vi "LinxSpiWriteRead.vi"(5 "CS Configuration":T1, 7 "SPI Channel":u8, 8 "Error In":errorcluster, 9 "SPI Frame Size (0)":u8, 10 "Data":u8[](array[numeric]), 11 "LINX Resource":T3) -> (0 "Error Out":errorcluster, 2 "Data":u8[](array[numeric]), 3 "LINX Resource":T3, 4 "status":i32)   [LabVIEW 2019, in "LMH-LINX.lvlib" / "Local IO.lvlib"]
uses:
  <vilib>/MakerHub/LINX/Private/Local IO/Local IO.lvlib
  <vilib>/MakerHub/LINX/Private/Type Defs/LINX Ref.ctl
  <vilib>/MakerHub/LINX/Private/Type Defs/Platform.ctl
  <vilib>/MakerHub/LINX/Private/Type Defs/Interface.ctl
  <vilib>/MakerHub/LINX/Private/Device/Type Defs/LINX Device Config.ctl
  <vilib>/MakerHub/LINX/Private/Device/Type Defs/TCP Config.ctl
  <vilib>/MakerHub/LINX/Private/Device/Type Defs/Channels.ctl
  <vilib>/MakerHub/LINX/Public/Peripherals/SPI/SPI CS Config.ctl
  <vilib>/MakerHub/LINX/Private/Type Defs/Peripherals/SPI/SPI CS Logic Level.ctl
  <vilib>/MakerHub/LINX/Private/Type Defs/Error Type.ctl
  <vilib>/MakerHub/LINX/LMH-LINX.lvlib
  <vilib>/MakerHub/LINX/Private/Type Defs/Channel FGV States.ctl
  <vilib>/myRIO/Common/Instrument Driver Framework/myRIO v1.0/SPI/typedefs/SPI Frame Length.ctl
  <vilib>/myRIO/Common/Instrument Driver Framework/myRIO v1.0/SPI/typedefs/SPI Data Direction.ctl
  <vilib>/myRIO/Common/Instrument Driver Framework/myRIO v1.0/SPI/typedefs/SPI Clock Polarity.ctl
  <vilib>/myRIO/Common/Instrument Driver Framework/myRIO v1.0/SPI/typedefs/SPI Clock Phase.ctl
  <vilib>/myRIO/Instrument Drivers/Onboard IO/SPI/typedefs/SPI Configuration.ctl
  <vilib>/myRIO/Common/Instrument Driver Framework/myRIO v1.0/SPI/typedefs/SPI Channels Enum.ctl
  <vilib>/myRIO/Common/Instrument Driver Framework/Utilities/typedefs/Generic FPGA Reference.ctl
  <vilib>/myRIO/Common/Instrument Driver Framework/Utilities/typedefs/myRIO v1.0 Reference.ctl
  <vilib>/myRIO/Common/Instrument Driver Framework/Utilities/typedefs/Hardware Version Enum.ctl
  <vilib>/myRIO/Common/Instrument Driver Framework/Utilities/typedefs/myRIO Generic Hardware Reference.ctl
  <vilib>/myRIO/Instrument Drivers/Onboard IO/SPI/typedefs/SPI Reference.ctl
  <vilib>/MakerHub/LINX/Resources/liblinxdevice.dll
  <vilib>/MakerHub/LINX/Private/Device/Device.lvlib
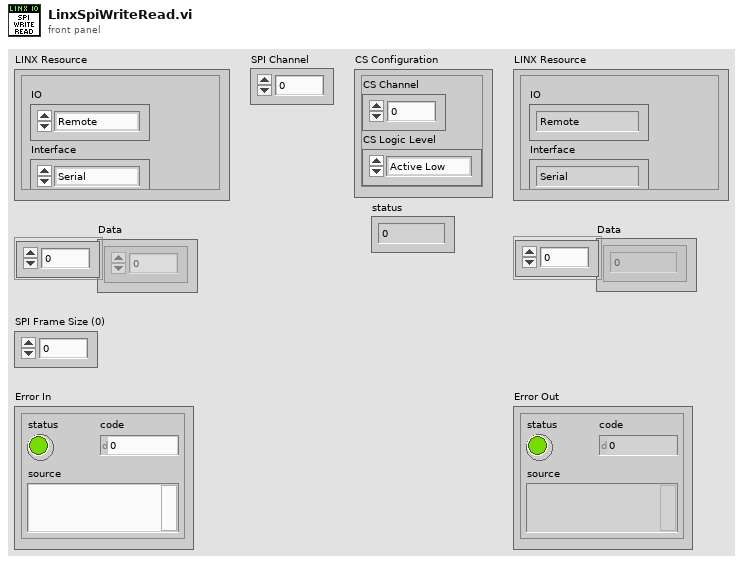
[diagram p1: front panel]
types:
  T1 = typedef "LMH-LINX.lvlib/SPI CS Config.ctl" = cluster{"CS Channel":u8, "CS Logic Level":T2}
  T2 = typedef "LMH-LINX.lvlib/SPI CS Logic Level.ctl" = enum8{"Active Low", "Active High"}
  T3 = typedef "LMH-LINX.lvlib/LINX Ref.ctl" = cluster{"IO":T4, "Interface":T5, "LINX Device Config":T6}
  T4 = typedef "LMH-LINX.lvlib/Platform.ctl" = enum16{"Remote", "Local"}
  T5 = typedef "LMH-LINX.lvlib/Interface.ctl" = enum16{"Serial", "TCP"}
  T6 = typedef "LMH-LINX.lvlib/Device.lvlib/LINX Device Config.ctl" = cluster{"Interface":T5, "COM Port":refnum<visa-resource-name>, "TCP Configuration":T7, "Device Family":u8, "Device ID":u8, "Device Name":string, "TCP Ref":refnum<k5>, "Channels":T8}
  T7 = typedef "LMH-LINX.lvlib/Device.lvlib/TCP Config.ctl" = cluster{"IP Address":string, "Port":u16}
  T8 = typedef "LMH-LINX.lvlib/Channels.ctl" = cluster{"DI":u8[], "DO":u8[], "AI":u8[], "AO":u8[], "PWM":u8[], "QE":u8[], "UART":u8[], "I2C 2":u8[], "SPI":u8[], "CAN":u8[], "Servo":u8[], "AI Ref (V)":dbl, "AI Resolution (Bits)":u8, "AO Ref (V)":dbl, "AO Resolution (Bits)":u8}
  T9 = typedef "LMH-LINX.lvlib/Error Type.ctl" = enum16{"Unknown", "Timeout", "Corrupt Return Packet", "Unable To Connect", "Command Not Supported", "Channel DNE", "Invalid COM Config", "Firmware Version Mismatch", "myRIO Support", "CMD Specific Error", "Local IO Not Supported"}
  T10 = typedef "LMH-LINX.lvlib/Channel FGV States.ctl" = enum16{"Initialize", "Get", "Set"}
  T11 = typedef "SPI.lvlib/SPI Reference.ctl" = cluster{"myRIO Reference":T12, "SPI Channels Enum":T16, "SPI Configuration":T17}
  T12 = typedef "myRIO Generic Hardware Reference.ctl" = cluster{"myRIO Model":T13, "myRIO Hardware Reference":T14}
  T13 = typedef "Hardware Version Enum.ctl" = enum16{"Unknown", "myRIO-1900", "myRIO-1950"}
  T14 = typedef "myRIO v1.0 Reference.ctl" = cluster{"Generic FPGA Reference":T15, "Allow multiple opens":bool}
  T15 = typedef "Generic FPGA Reference.ctl" = refnum<k20>
  T16 = typedef "SPI Channels Enum.ctl" = enum16{"Not Connected", "A/SPI", "B/SPI"}
  T17 = typedef "SPI.lvlib/SPI Configuration.ctl" = cluster{"Frequency [Hz]":dbl, "Clock Phase":T18, "Clock Polarity":T19, "Data Direction":T20, "Frame Length":T21}
  T18 = typedef "SPI Clock Phase.ctl" = enum8{"Leading", "Trailing"}
  T19 = typedef "SPI Clock Polarity.ctl" = enum8{"Low", "High"}
  T20 = typedef "SPI Data Direction.ctl" = enum8{"Most significant bit first", "Least significant bit first"}
  T21 = typedef "SPI Frame Length.ctl" = u8
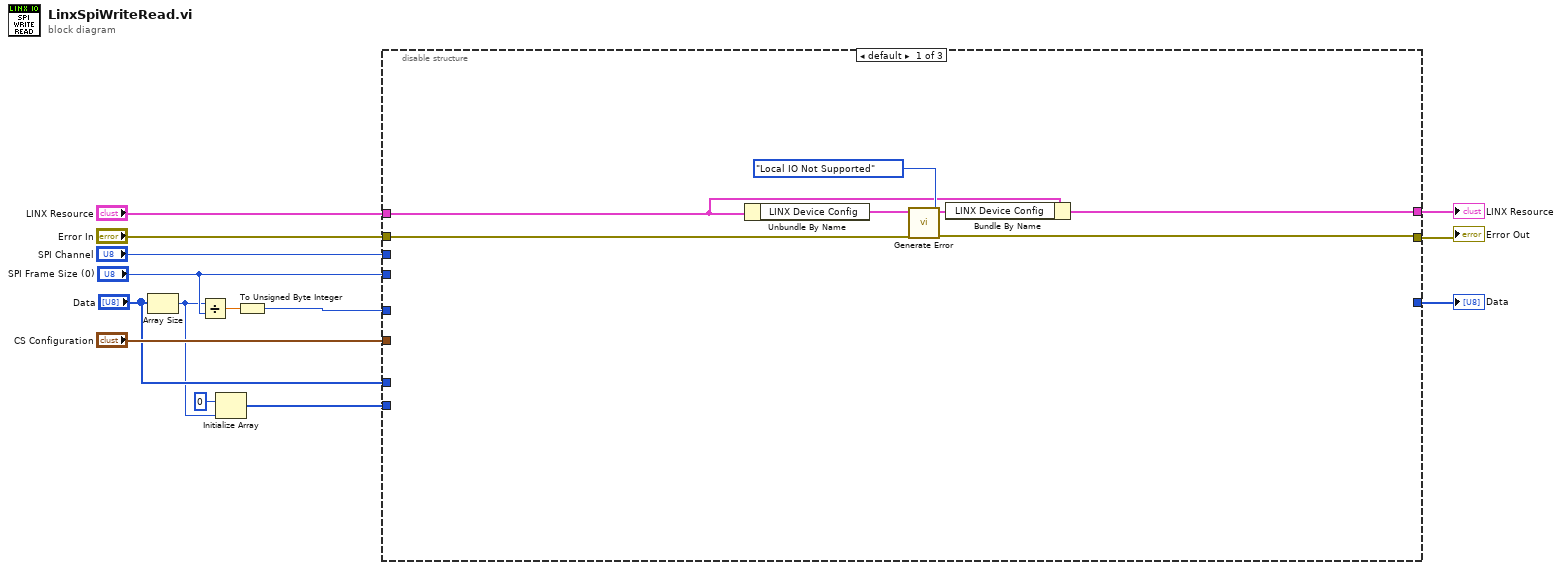
[diagram p0: block diagram]
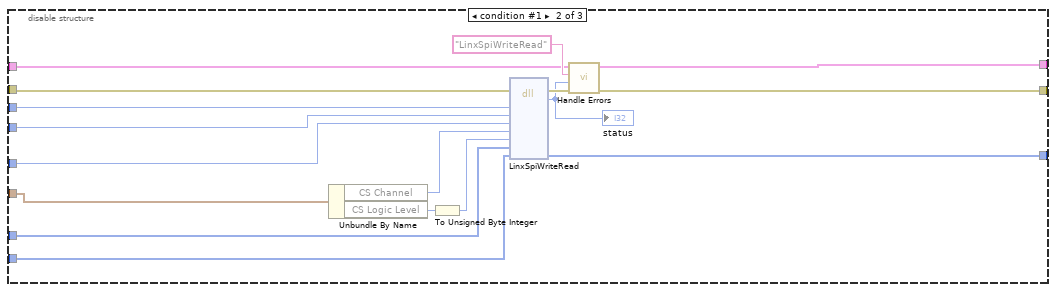
[diagram p2: hidden frame]
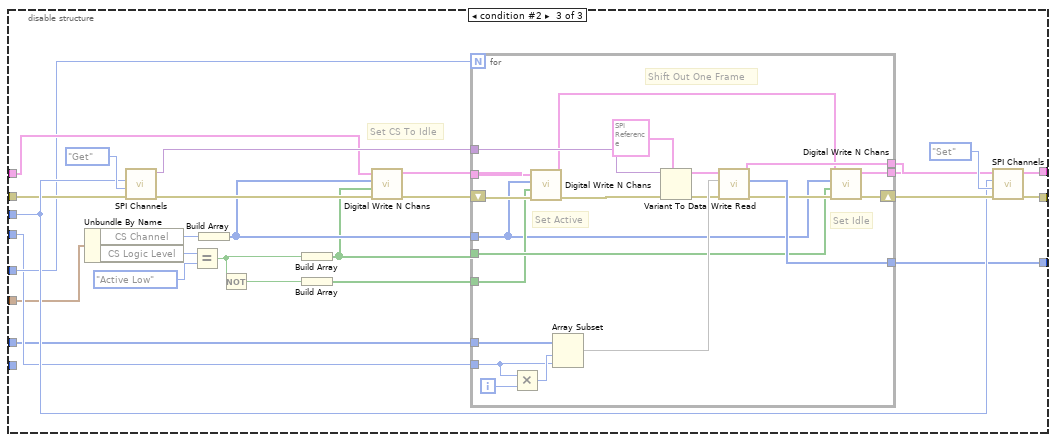
[diagram p3: hidden frame]
diagram:
  n1 = Array Size(array="Data") -> (size(s)=w4:i32)
  n2 = Divide(x=w4, y="SPI Frame Size (0)") -> (x/y=w7:dbl)
  n3 = Initialize Array(u8 0 ("element"), w4) -> (w2:u8[])
  n4 = To Unsigned Byte Integer(number=w7) -> (unsigned 8bit integer=w6:u8)
  n5 = disable-structure shown="default" {
    disable-tunnel: [w16 w23 w41] -> w14
    disable-tunnel: "LINX Resource" -> [w18 w33 w48]
    disable-tunnel: "Error In" -> [w20 w36 w49]
    disable-tunnel: "SPI Channel" -> [_ w34 w50]
    disable-tunnel: [w15 w24 w40] -> w10
    disable-tunnel: "SPI Frame Size (0)" -> [_ w32 w46]
    disable-tunnel: w6 -> [_ w30 w47]
    disable-tunnel: "CS Configuration" -> [_ w31 w44]
    disable-tunnel: "Data" -> [_ w26 w45]
    disable-tunnel: w2 -> [_ w25 _]
    disable-tunnel: [_ w22 w39] -> w1
    frame condition #0 (active) {
      n6 = Unbundle By Name(w18) -> ("LINX Device Config"=w19:T6)
      n7 = call <vilib>:"Generate Error.vi"("Error In"=w20, "Error Type"=Error_Type."Local IO Not Supported", "LINX Device Config"=w19) -> ("Error Out"=w15:errorcluster, "Dup LINX Device Config"=w17:T6)  [unwired: 7 in]
      n8 = Bundle By Name(cluster=w18, "LINX Device Config"=w17) -> (w16:T3)
    }
    frame condition #1 {
      n9 = Unbundle By Name(w31) -> ("CS Channel"=w29:u8, "CS Logic Level"=w28:T2)
      n10 = To Unsigned Byte Integer(number=w28) -> (unsigned 8bit integer=w27:u8)
      n11 = dll-call lib="E:/lv2019/dist/vi.lib/MakerHub/LINX/Resources/liblinxdevice.*" fn="LinxSpiWriteRead"(error in=w36, "channel"=w34, "frameSize"=w32, "numFrames"=w30, "csChan"=w29, "csLL"=w27, "sendBuffer"=w26, "recBuffer"=w25) -> (error out=w37:errorcluster, "status"=w35:i32, "recBuffer"=w22:u8[])  [unwired: 8 in, 1 out]
      "status" <- w35
      n12 = call <vilib>:"Handle Errors.vi"("Error In"=w37, "LinxStatus"=w35, "Function Name"="LinxSpiWriteRead", "LINX Resource"=w33) -> ("Error Out"=w24:errorcluster, "LINX Resource"=w23:T3)  [unwired: 6 in]
    }
    frame condition #2 {
      # "Set CS To Idle"
      n13 = Unbundle By Name(w44) -> ("CS Channel"=w43:u8, "CS Logic Level"=w42:T2)
      n14 = call <vilib>:"SPI Channels.vi"("Error In"=w49, "Channel State"=Channel_FGV_States."Get", "Channel Number"=w50) -> ("Error Out"=w59:errorcluster, "SPI Channel"=w60:variant)  [unwired: 7 in]
      n15 = Equal?(x=w42, y=SPI_CS_Logic_Level."Active Low") -> (x = y?=w54:bool)
      n16 = Build Array(w43) -> (w55:u8[])
      n17 = Not(x=w54) -> (.not. x?=w52:bool)
      n18 = Build Array(w54) -> (w53:bool[])
      n19 = Build Array(w52) -> (w51:bool[])
      n20 = call <vilib>:"Digital Write N Chans.vi"("Error In"=w59, "Values"=w53, "DO Channels"=w55, "LINX Resource"=w48) -> ("Error Out"=w58:errorcluster, "LINX Resource"=w56:T3)  [unwired: 6 in]
      n21 = for {
        N: w47 -> [_]
        tunnel: [w85] -> w61
        tunnel: w60 -> [w84]
        tunnel: w45 -> [w82]
        tunnel: [w83] -> w39
        shift-right: [w74] -> w62
        shift-left: w58 -> [w77]
        tunnel: w46 -> [w78]
        tunnel: w56 -> [w75]
        tunnel: w55 -> [w68]
        tunnel: [w71] -> w41
        tunnel: w53 -> [w70]
        tunnel: w51 -> [w69]
        i -> [w80]
        # "Set Idle"
        # "Shift Out One Frame"
        # "Set Active"
        n22 = Multiply(x=w78, y=w80) -> (x*y=w79:i32)
        n23 = call <vilib>:"Digital Write N Chans.vi"("Error In"=w77, "Values"=w69, "DO Channels"=w68, "LINX Resource"=w75) -> ("Error Out"=w76:errorcluster, "LINX Resource"=w72:T3)  [unwired: 6 in]
        n24 = Array Subset(array=w82, index=w79, length=w78) -> (w81:u8[])
        n25 = Variant To Data(error in=w76, type=T11 {"myRIO Reference"={"myRIO Model"=enum."Unknown", "myRIO Hardware Reference"={"Generic FPGA Reference"=refnum, "Allow multiple opens"=FALSE}}, "SPI Channels Enum"=enum."Not Connected", "SPI Configuration"={"Frequency [Hz]"=0.0, "Clock Phase"=enum."Leading", "Clock Polarity"=enum."Low", "Data Direction"=enum."Most significant bit first", "Frame Length"=8}} ("SPI Ref In"), Variant=w84) -> (data=w66:T11, error out=w65:errorcluster)
        n26 = call <vilib>:"Write Read.vi"("error in (no error)"=w65, "Frames to Write"=w81, "SPI Ref In"=w66) -> ("error out"=w73:errorcluster, "Frames Read"=w83:u16[], "SPI Ref Out"=w85:T11)  [unwired: 6 in]
        n27 = call <vilib>:"Digital Write N Chans.vi"("Error In"=w73, "Values"=w70, "DO Channels"=w68, "LINX Resource"=w72) -> ("Error Out"=w74:errorcluster, "LINX Resource"=w71:T3)  [unwired: 6 in]
      }
      n28 = call <vilib>:"SPI Channels.vi"("Error In"=w62, "Channel State"=Channel_FGV_States."Set", "Channel Number"=w50, "SPI Channel"=w61) -> ("Error Out"=w40:errorcluster)  [unwired: 6 in, 1 out]
    }
  }
  "LINX Resource" <- w14
  "Error Out" <- w10
  "Data" <- w1
